vi "Vision Research Phantom Series PhCon PhComputeWB.vi"(1 "pP":T3, 2 "SquareSide":i32, 3 "pPixel":u16[](array[numeric]), 5 "Error In (no error)":errorcluster, 6 "BITMAPINFOHEADER":T4, 7 "CFA":T1 {"CFA" items=["CFA_NONE", "CFA_VRI", "CFA_VRIV6", "CFA_BAYER", "CFA_BAYERFLIP"]}) -> (14 "WBGAIN":T2, 15 "pSatCnt":u32, 16 "pPixel out":u16[](array[numeric]), 19 "Error Out":errorcluster)   [LabVIEW 2013, in "VRI.lvlib"]
doc: "PhCon.dll\n\nPhComputeWB\nHRESULT PhComputeWB(PBITMAPINFOHEADER pBMIH, PBYTE pPixel, PPOINT pP, int SquareSide, \nUINT CFA, PWBGAIN pWB, PUINT pSatCnt)\n\nParameters Description\npBMIH (in) Image header.\npPixel (in) Image pixels.\npP (in) Point to compute the WB around.\nSquareSide (in) Square side of the area to compute WB.\nCFA (in) Color filter array code of the sensor.\npWB (out) Result: WBGAIN, the compensating gains on red and blue (can be NULL if not\n needed).\npSatCnt (out) Saturated pixels count (can be NULL if not needed).\nReturn HRESULT (0 = Ok)\nComments Computes the compensating WBGAIN based on the pixels color in the square \n specified by the center point and the side length.\n It is called from PhMeasureWB and can be also used for computing the White\n balance compensation gains when viewing a cine from camera or from file."
uses:
  VRI.lvlib
  _Type Defs/BITMAPINFOHEADER.ctl
  _Type Defs/Point.ctl
  _Type Defs/PhInt WBGAIN.ctl
  _Type Defs/PhInt CFA.ctl
  Phantom DLLs/PhCon.Dll
panel:
  # "For instructions on the use of this VI, press Ctrl+H to display the help window and move the mouse over the icon, controls, and indicators"
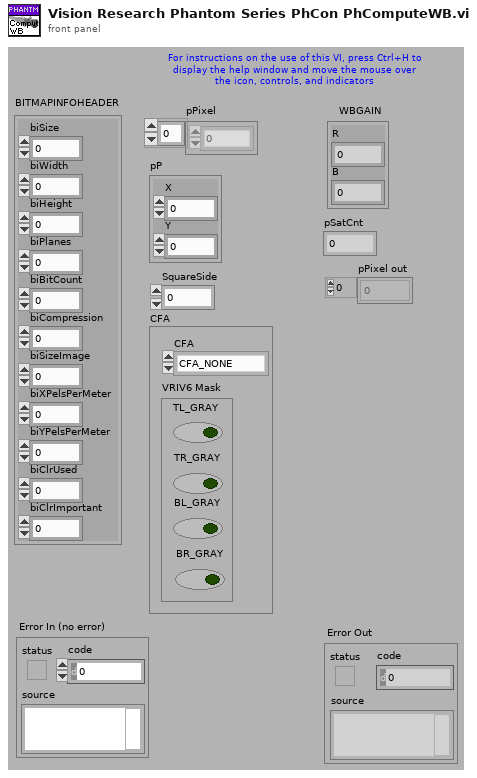
[diagram p1: front panel]
types:
  T1 = typedef "VRI.lvlib/PhInt CFA.ctl" = cluster{"CFA":u32, "VRIV6 Mask":cluster{"TL_GRAY":bool, "TR_GRAY":bool, "BL_GRAY":bool, "BR_GRAY":bool}}
  T2 = typedef "VRI.lvlib/PhInt WBGAIN.ctl" = cluster{"R":sgl, "B":sgl}
  T3 = typedef "VRI.lvlib/Point.ctl" = cluster{"X":i32, "Y":i32}
  T4 = typedef "VRI.lvlib/BITMAPINFOHEADER.ctl" = cluster{"biSize":u32, "biWidth":i32, "biHeight":i32, "biPlanes":u16, "biBitCount":u16, "biCompression":u32, "biSizeImage":u32, "biXPelsPerMeter":i32, "biYPelsPerMeter":i32, "biClrUsed":u32, "biClrImportant":u32}
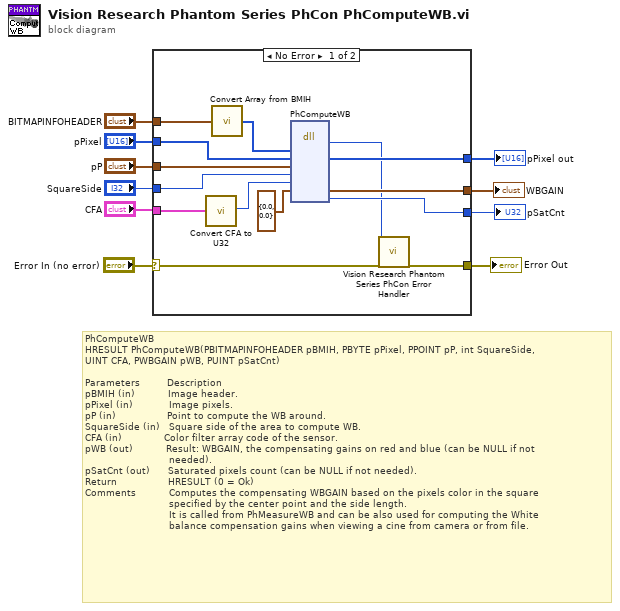
[diagram p0: block diagram]
diagram:
  # "PhComputeWB\nHRESULT PhComputeWB(PBITMAPINFOHEADER pBMIH, PBYTE pPixel, PPOINT pP, int SquareSide, \nUINT CFA, PWBGAIN pWB, PUINT pSatCnt)\n\nParameters         Description\npBMIH (in)           Image header.\npPixel (in)            Image pixels.\npP (in)                 Point to compute the WB around.\nSquareSide (in)   Square side of the area to compute WB.\nCFA (in)              Color filter array code of the sensor.\npWB (out)           Result: WBGAIN, the compensating gains on red and blue (can be NULL if not\n                            needed).\npSatCnt (out)      Saturated pixels count (can be NULL if not needed).\nReturn                 HRESULT (0 = Ok)\nComments           Computes the compensating WBGAIN based on the pixels color in the square \n                            specified by the center point and the side length.\n                            It is called from PhMeasureWB and can be also used for computing the White\n                            balance compensation gains when viewing a cine from camera or from file."
  n1 = case shown="No Error" "Error In (no error)" {
    selector: "Error In (no error)" -> [w24 w25]
    tunnel: [w23 w25] -> w9
    tunnel: "BITMAPINFOHEADER" -> [w22 _]
    tunnel: "pPixel" -> [w21 _]
    tunnel: "pP" -> [w20 _]
    tunnel: "SquareSide" -> [w19 _]
    tunnel: "CFA" -> [w18 _]
    tunnel: [w17 _] -> w4
    tunnel: [w16 _] -> w3
    tunnel: [w15 _] -> w1
    frame No Error {
      n2 = call "Convert CFA to U32.vi"("CFA in"=w18) -> ("CFA out"=w11:u32)  [unwired: 18 out]
      n3 = call "Convert Array from BMIH.vi"("BITMAPINFOHEADER"=w22) -> ("Array"=w13:u8[])
      n4 = dll-call lib="C:/Projects/SDK/64-bit/Vision Research Phantom Series Labview Driver/Phantom DLLs/PhCon.dll" fn="PhComputeWB"("pBMIH"=w13, "pPixel"=w21, "pP"=w20, "SquareSide"=w19, "CFA"=w11, "pWB"=T2 {"R"=0.0, "B"=0.0} ("WBGAIN")) -> ("HRESULT"=w14:i32, "pPixel"=w15:u16[], "pWB"=w17:T2, "pSatCnt"=w16:u32)  [unwired: 7 in, 3 out]
      n5 = call "Vision Research Phantom Series PhCon Error Handler.vi"("ErrNo"=w14, "Error In (no error)"=w24) -> ("Error Out"=w23:errorcluster)  [unwired: 17 out]
    }
    frame Error {
    }
  }
  "Error Out" <- w9
  "WBGAIN" <- w4
  "pSatCnt" <- w3
  "pPixel out" <- w1
